vi "write TBM configuration.vi"(8 "error in":errorcluster, 10 "configuration":refnum<class "TBM configuration.lvclass">, 11 "Temperature Controller Logic editor node in":refnum<class "Temperature Controller Logic editor node.lvclass">) -> (0 "error out":errorcluster, 3 "Temperature Controller Logic editor node out":refnum<class "Temperature Controller Logic editor node.lvclass">)   [LabVIEW 2013, in "Temperature Controller Logic editor node.lvclass"]
uses:
  Temperature Controller Logic editor node.lvclass
  <vilib>/NI/Tag Bus Module Framework/root configuration/TBM configuration.lvclass
  module/configuration/Temperature Controller Logic configuration.lvclass
  Temperature Controller Logic editor node.lvclass/Temperature Controller Logic editor node.ctl
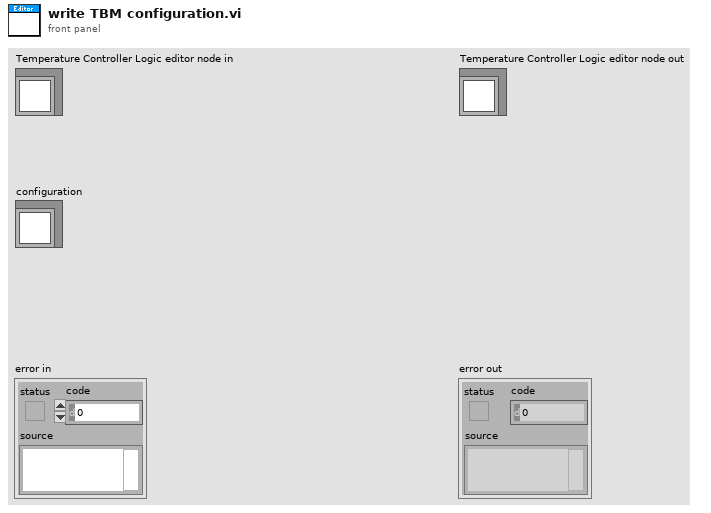
[diagram p1: front panel]
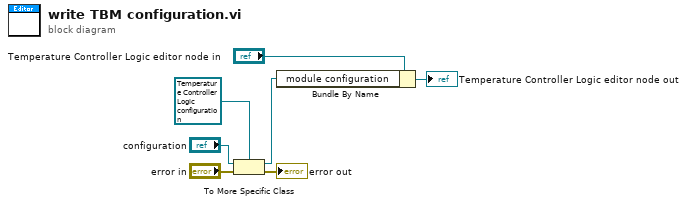
[diagram p0: block diagram]
diagram:
  n1 = To More Specific Class(target class=refnum<class "Temperature Controller Logic configuration.lvclass"> refnum ("module configuration"), reference="configuration", error in="error in") -> (specific class reference=w1:refnum<class "Temperature Controller Logic configuration.lvclass">, error out=→"error out":errorcluster)
  n2 = Bundle By Name(cluster="Temperature Controller Logic editor node in", "module configuration"=w1) -> (→"Temperature Controller Logic editor node out":refnum<class "Temperature Controller Logic editor node.lvclass">)
